vi "生成ID号数据.vi"(11 "字符串":string="12354678") -> (3 "ID代码":u8[](array[numeric]) format="%x")   [LabVIEW 2015]
panel:
  out "大小":i32
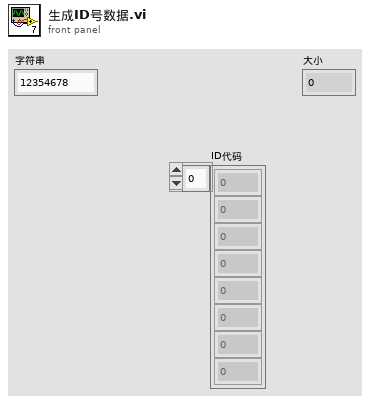
[diagram p1: front panel]
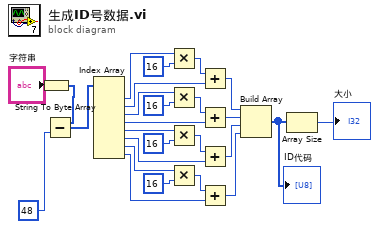
[diagram p0: block diagram]
diagram:
  n1 = String To Byte Array(string="字符串") -> (unsigned byte array=w3:u8[])
  n2 = Subtract(x=w3, y=48) -> (x-y=w2:i32[])
  n3 = Index Array(array=w2) -> (element #1=w24:i32, element #2=w21:i32, element #3=w19:i32, element #4=w18:i32, element #5=w15:i32, element #6=w14:i32, element #7=w11:i32, element #8=w10:i32)  [unwired: 8 in]
  n4 = Multiply(x=w24, y=u8 16) -> (x*y=w22:i32)
  n5 = Multiply(x=w19, y=u8 16) -> (x*y=w8:i32)
  n6 = Multiply(x=w15, y=u8 16) -> (x*y=w16:i32)
  n7 = Multiply(x=w11, y=u8 16) -> (x*y=w12:i32)
  n8 = Add(x=w22, y=w21) -> (x+y=w9:i32)
  n9 = Add(x=w8, y=w18) -> (x+y=w6:i32)
  n10 = Add(x=w16, y=w14) -> (x+y=w7:i32)
  n11 = Add(x=w12, y=w10) -> (x+y=w5:i32)
  n12 = Build Array(w9, w6, w7, w5) -> (w4:i32[])
  "ID代码" <- w4
  n13 = Array Size(array=w4) -> (size(s)=→"大小":i32)
